vi "Generate Event.vi"(8 "error in (no error)":errorcluster, 10 "Event Data":cluster{"Event":string, "Data":variant}) -> (0 "error out":errorcluster)   [LabVIEW 2023, in "Template.lvlib"]
uses:
  Template.lvlib
  Events/Controls/FGV Event State.ctl
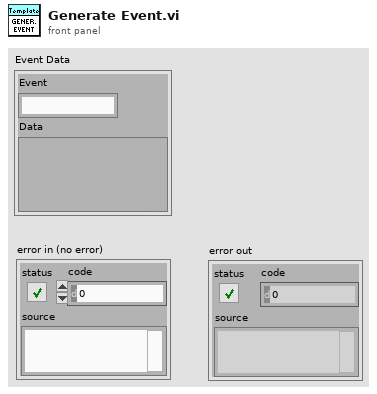
[diagram p1: front panel]
types:
  T1 = typedef "FGV Event State.ctl" = enum16{"Get", "Set"}
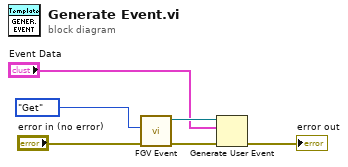
[diagram p0: block diagram]
diagram:
  n1 = call "FGV Event.vi"("error in (no error)"="error in (no error)", "FGV Event State"=FGV_Event_State."Get") -> ("error out"=w2:errorcluster, "user event out"=w4:refnum<user-event>)  [unwired: 8 in]
  n2 = Generate User Event(user event=w4, event data cluster="Event Data", error in=w2) -> (error out=→"error out":errorcluster)  [unwired: 1 in, 1 out]
